vi "TLS Server.vi"() -> ()   [LabVIEW 2020, in "Test.lvlib"]
uses:
  Test.lvlib
  TCP Comms/TinyTCP.lvlib
  2a5d5669-415a-424a-977b-6d88a7b7cc3d.vi
  TCP Comms/Cert Chain.ctl
  TCP Comms/Server TLS Config.ctl
  4b3f1b52-7145-433c-ac39-6bfb55dfd7bc.vi
  Client Data.ctl
  TCP Comms/State.ctl
  Server Data.ctl
panel:
  out "Client Data":T1 {"Slide" scale=0.0..10.0}
  in  "Server Data":T2
  out "Error":errorcluster
  in  "Close":bool
  in  "Open":bool
  out "Server State":T3
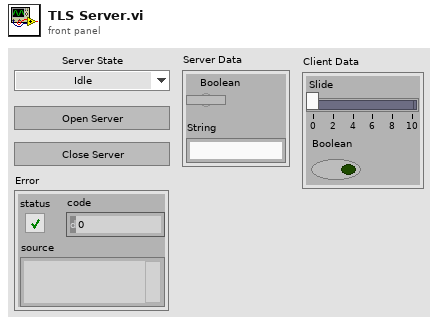
[diagram p1: front panel]
types:
  T1 = typedef "Test.lvlib/Client Data.ctl" = cluster{"Slide":dbl, "Boolean":bool}
  T2 = typedef "Test.lvlib/Server Data.ctl" = cluster{"Boolean":bool, "String":string}
  T3 = typedef "TinyTCP.lvlib/State.ctl" = enum16{"Idle", "Starting", "Connecting", "Connected", "Disconnecting", "Stopped"}
  T4 = typedef "TinyTCP.lvlib/Server TLS Config.ctl" = cluster{"Private Key Path":path, "Private Key Format":enum32{"PKCS#8 (PEM)", "PKCS#8 (DER)"}, "Password":string, "Cert Chain":T5}
  T5 = typedef "TinyTCP.lvlib/Cert Chain.ctl" = cluster{"Path":path, "Format":enum32{"X.509 (PEM)"}}
  T6 = typedef "TinyTCP.lvlib/Instance.ctl" = refnum<data-value>
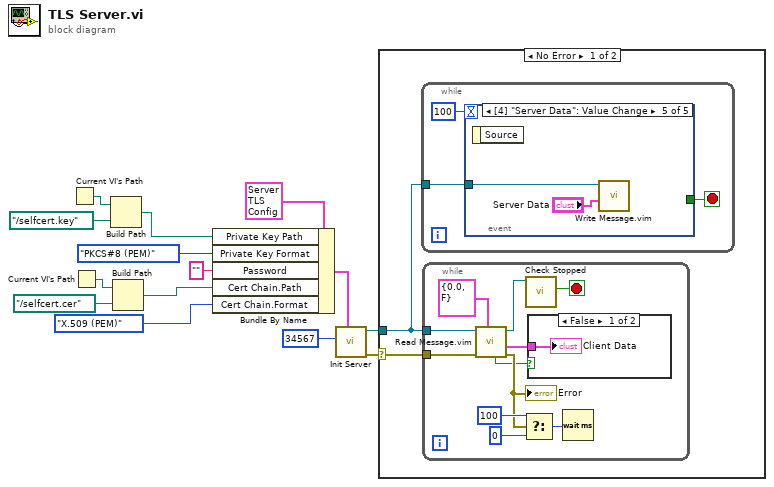
[diagram p0: block diagram]
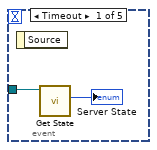
[diagram p3: hidden frame]
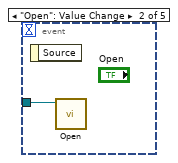
[diagram p4: hidden frame]
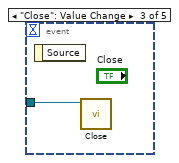
[diagram p5: hidden frame]
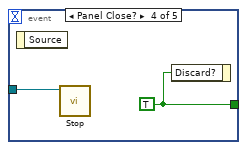
[diagram p6: hidden frame]
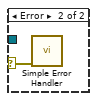
[diagram p7: hidden frame]
diagram:
  n1 = Current VI's Path() -> (path=w9:path)
  n2 = Current VI's Path() -> (path=w4:path)
  n3 = Build Path(base path=w9, name or relative path=path "../selfcert.key") -> (appended path=w7:path)
  n4 = Build Path(base path=w4, name or relative path=path "../selfcert.cer") -> (appended path=w2:path)
  n5 = Bundle By Name(cluster=T4 {"Private Key Path"=path "", "Private Key Format"=enum."PKCS#8 (PEM)", "Password"="", "Cert Chain"={"Path"=path "", "Format"=enum."X.509 (PEM)"}} ("Server TLS Config"), "Private Key Path"=w7, "Private Key Format"=enum32{"PKCS#8 (PEM)", "PKCS#8 (DER)"}."PKCS#8 (PEM)", "Password"="", "Cert Chain.Path"=w2, "Cert Chain.Format"=enum32{"X.509 (PEM)"}."X.509 (PEM)" ("Format")) -> (w11:T4)
  n6 = call "Init Server.vi"("Server TLS Config (Disabled)"=w11, "Port"=u16 34567) -> ("error out"=w14:errorcluster, "TinyTCP Server"=w10:T6)  [unwired: 8 in]
  n7 = case shown="No Error" w14 {
    selector: w14 -> [w16 w40]
    tunnel: w10 -> [w15 _]
    frame No Error {
      n8 = while {
        tunnel: w15 -> [w31]
        stop <- w30 stop-if-true
        n9 = event shown="[4] \"Server Data\": Value Change" {
          selector: _ -> [_ _ _ _ _]
          dyn-events: _ -> [_ _ _ _ _]
          timeout: 100 -> [_ _ _ _ _]
          tunnel: w31 -> [w33 w34 w35 w37 w39]
          tunnel: [_ _ _ w36 _] -> w30
          event Timeout {
            n10 = event-data() -> ()  [unwired: 1 in, 1 out]
            n11 = call "Get State.vi"("TCP Comm In"=w33) -> ("State"=→"Server State":T3)  [unwired: 9 in, 1 out]
          }
          event "Open": Value Change {
            n12 = event-data() -> ()  [unwired: 1 in, 1 out]
            n13 = call "Open.vi"("TCP Comm"=w34) -> ()  [unwired: 10 in, 1 out]
          }
          event "Close": Value Change {
            n14 = event-data() -> ()  [unwired: 1 in, 1 out]
            n15 = call "Close.vi"("TCP Comm"=w35) -> ()  [unwired: 10 in, 1 out]
          }
          event Panel Close? {
            w36 = TRUE
            n16 = event-data() -> ()  [unwired: 1 in, 1 out]
            n17 = call "Stop.vi"("TCP Comm"=w37) -> ()  [unwired: 10 in, 1 out]
            n18 = event-data("Discard?"=w36) -> ()  [unwired: 1 in, 1 out]
          }
          event Value Change {
            n19 = event-data() -> ()  [unwired: 1 in, 1 out]
            n20 = call "Write Message.vim"("Data"="Server Data", "TCP Comm In"=w39) -> ()  [unwired: 7 in, 3 out]
          }
        }
      }
      n21 = while {
        tunnel: w15 -> [w18]
        tunnel: w16 -> [w27]
        stop <- w22 stop-if-true
        n22 = call "Read Message.vim"("Data Type (Raw Data)"=T1 {"Slide"=0.0, "Boolean"=FALSE} ("Client Data"), "error in (no error)"=w27, "TCP Comm In"=w18) -> ("error out"=w21:errorcluster, "Data"=w20:T1, "TCP Comm"=w23:T6, "Timeout?"=w19:bool)  [unwired: 3 in, 2 out]
        "Error" <- w21
        n23 = Select(t=u32 100, s=w21, f=u32 0 ("milliseconds to wait")) -> (s? t:f=w25:u32)
        n24 = call "Check Stopped.vi"("TCP Comm In"=w23) -> ("Stopped?"=w22:bool)  [unwired: 9 in, 1 out]
        n25 = case shown="False" w19 {
          tunnel: w20 -> [w28 _]
          frame False {
            "Client Data" <- w28
          }
          frame True {
          }
        }
        n26 = Wait (ms)(milliseconds to wait=w25) -> ()  [unwired: 1 out]
      }
    }
    frame Error {
      n27 = call <vilib>:"Simple Error Handler.vi"("error in (no error)"=w40) -> ()  [unwired: 4 in, 5 out]
    }
  }
